vi "Conditional Disable Structrue.vi"() -> ()   [LabVIEW 2020]
panel:
  out "Output":i32[](array[numeric])
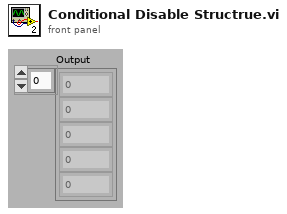
[diagram p1: front panel]
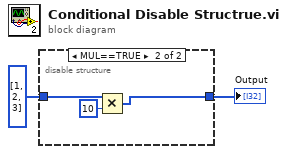
[diagram p0: block diagram]
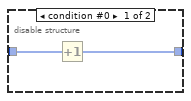
[diagram p2: hidden frame]
diagram:
  n1 = disable-structure shown="MUL==TRUE" {
    disable-tunnel: i32[] [1, 2, 3] -> [w4 w7]
    disable-tunnel: [w3 w5] -> w1
    frame condition #0 {
      n2 = Increment(x=w4) -> (x+1=w3:i32[])
    }
    frame condition #1 (active) {
      n3 = Multiply(x=w7, y=10) -> (x*y=w5:i32[])
    }
  }
  "Output" <- w1
